vi "SS_FPGA_Drop1_all_in_v3.vi"() -> ()   [LabVIEW 2016]
uses:
  <vilib>/rvi/Emulation/niFpgaGetClockAttributes.vi
  <vilib>/rvi/Emulation/niFpgaSctlEmulationGetInTimedLoop.vi
  <vilib>/rvi/Emulation/niFpgaEmulationReportErrorSimple.vi
  <vilib>/rvi/Emulation/niFpgaCriticalErrorInLSC.vi
  <vilib>/rvi/Emulation/niFpgaProcessEmulError.vi
  <vilib>/rvi/eio/common/nirviEmuTemplateMethod_errors.vi
  <vilib>/eio/EIONode/EIONode.xnode
  <vilib>/rvi/FXPMathLib/FxpMul/XNode/nifxpmath_Multiplier.xnode
  <vilib>/rvi/FXPMathLib/FxpAdd/XNode/nifxpmath_Add.xnode
  <vilib>/rvi/FXPMathLib/sim/FxpSim.dll
panel:
  in  "Tab Control":T1(tab)
  in  "Start Acquisition":bool
  out "Actual Duration (ms)":u32
  out "Number of Loop 1 Samples":i32
  in  "Scan Rate (mSec) Loop 1":u32 caption="Count(mSec)"
  in  "Reset":bool
  in  "FSIS Interlock":bool
  out "Raw Data In Mod 1":fxp<+,24,12>[](array[numeric])
  in  "offset mod 1":fxp<+,24,12>[](array[numeric])=[0.0, 0.0, 0.0, 0.0, 0.0, 0.0, 0.0, 0.0, 0.0, 0.0, 0.0, 0.0, 0.0, 0.0, 0.0, 0.0]
  in  "cal mod 1":fxp<+,24,12>[](array[numeric])=[10.0, 10.0, 10.0, 10.0, 10.0, 10.0, 10.0, 10.0, 10.0, 10.0, 10.0, 10.0, 10.0, 10.0, 10.0, 10.0]
  out "Cal value out Mod 1":fxp<+,24,12>[](array[numeric]) format="%.16g"
  out "PTF - No Operations Mod 1":bool[](array[boolean])
  in  "lower limit \nNOOP mod 1":fxp<+,24,12>[](array[numeric])=[0.0, 0.0, 0.0, 0.0, 0.0, 0.0, 0.0, 0.0, 0.0, 0.0, 0.0, 0.0, 0.0, 0.0, 0.0, 0.0]
  in  "upper limit \nOKOP mod 1":fxp<+,24,12>[](array[numeric])=[0.0, 0.0, 0.0, 0.0, 0.0, 0.0, 0.0, 0.0, 0.0, 0.0, 0.0, 0.0, 0.0, 0.0, 0.0, 0.0]
  out "PTF - Warning Mod 1":bool[](array[boolean])
  in  "NOOPS Fault Filter mod 1":u16[](array[numeric])=[0, 0, 0, 0, 0, 0, 0, 0, 0, 0, 0, 0, 0, 0, 0, 0]
  out "Raw Data In Mod 2":fxp<+,24,12>[](array[numeric]) format="%.27g"
  in  "offset mod 2":fxp<+,24,12>[](array[numeric])=[0.0, 0.0, 0.0, 0.0, 0.0, 0.0, 0.0, 0.0, 0.0, 0.0, 0.0, 0.0, 0.0, 0.0, 0.0, 0.0]
  in  "cal mod 2":fxp<+,24,12>[](array[numeric])=[0.0, 0.0, 0.0, 0.0, 0.0, 0.0, 0.0, 0.0, 0.0, 0.0, 0.0, 0.0, 0.0, 0.0, 0.0, 0.0]
  out "PTF - No Operations Mod 2":bool[](array[boolean])
  in  "lower limit \nNOOP mod 2":fxp<+,24,12>[](array[numeric])=[0.0, 0.0, 0.0, 0.0, 0.0, 0.0, 0.0, 0.0, 0.0, 0.0, 0.0, 0.0, 0.0, 0.0, 0.0, 0.0]
  in  "upper limit \nOKOP mod 2":fxp<+,24,12>[](array[numeric])=[0.0, 0.0, 0.0, 0.0, 0.0, 0.0, 0.0, 0.0, 0.0, 0.0, 0.0, 0.0, 0.0, 0.0, 0.0, 0.0]
  out "Cal value out Mod 2":fxp<+,24,12>[](array[numeric])
  out "PTF - Warning Mod 2":bool[](array[boolean])
  in  "NOOPS Fault Filter mod 2":u16[](array[numeric])=[0, 0, 0, 0, 0, 0, 0, 0, 0, 0, 0, 0, 0, 0, 0, 0]
  out "Raw Data In Mod 3":fxp<+,24,12>[](array[numeric]) format="%.27g"
  in  "cal mod 3":fxp<+,24,12>[](array[numeric])=[0.0, 0.0, 0.0, 0.0, 0.0, 0.0, 0.0, 0.0, 0.0, 0.0, 0.0, 0.0, 0.0, 0.0, 0.0, 0.0]
  in  "offset mod 3":fxp<+,24,12>[](array[numeric])=[0.0, 0.0, 0.0, 0.0, 0.0, 0.0, 0.0, 0.0, 0.0, 0.0, 0.0, 0.0, 0.0, 0.0, 0.0, 0.0]
  out "PTF - No Operations Mod 3":bool[](array[boolean])
  in  "lower limit\nNOOP mod 3":fxp<+,24,12>[](array[numeric])=[0.0, 0.0, 0.0, 0.0, 0.0, 0.0, 0.0, 0.0, 0.0, 0.0, 0.0, 0.0, 0.0, 0.0, 0.0, 0.0]
  in  "upper limit\nOKOP mod 3":fxp<+,24,12>[](array[numeric])=[0.0, 0.0, 0.0, 0.0, 0.0, 0.0, 0.0, 0.0, 0.0, 0.0, 0.0, 0.0, 0.0, 0.0, 0.0, 0.0]
  out "PTF - Warning Mod 3":bool[](array[boolean])
  out "Cal value out Mod 3":fxp<+,24,12>[](array[numeric])
  in  "NOOPS Fault Filter mod 3":u16[](array[numeric])=[0, 0, 0, 0, 0, 0, 0, 0, 0, 0, 0, 0, 0, 0, 0, 0]
  out "Raw Data In Mod 4":fxp<+,24,12>[](array[numeric]) format="%.27g"
  out "Raw Data In Mod 5":fxp<+,24,12>[](array[numeric]) format="%.27g"
  out "Raw Data In Mod 6":bool[](array[boolean])
  out "Trigger from Trigger Card (SYNC and ASYNC) (Euro1Slot15)":bool
  out "Main Trigger In":bool
  out "SYNC/ASYNC":bool
  out "Beam Prepare":bool
  out "Override":bool
  out "320 Open":bool
  out "320  Closed":bool
  out "400 Open":bool
  out "400 Open Closed":bool
  out "Calorimeter Left Gate Open":bool
  out "Calorimeter Left Gate Closed":bool
  out "320  Bypass Open":bool
  out "320 Bypass Closed":bool
  out "Calorimeter Right Gate Closed":bool
  out "HV Area Water":bool
  out "MAST Area Air":bool
  out "Calorimeter Right Gate Open":bool
  in  "Control FBIS 1kHZ":bool
  # "CHANNEL ID"
  # "1"
  # "SS Source Body Flow\n\nSS Source Body Temperature\n\nSS Grid 1 Flow\n\nSS Grid 1 Temperature\n\nSS Grid 2 Flow\n\nSS Grid 2 Temperature\n\nSS Grid 3 Flow\n\nSS Grid 3 Temperature\n\nSS Grid 4/1st Stage Neutraliser Flow\n\nSS Grid 4/1st Stage Neutraliser Temperature\n\nSS 2nd Stage Neutraliser Flow\n\nSS 2nd Stage Neutraliser Temperature\n\nSS PINI Backplate Flow\n\nSS PINI Backplate Temperature\n\nSS Duct Scraper Flow\n\nSS Duct Scraper Temperature"
  # "2"
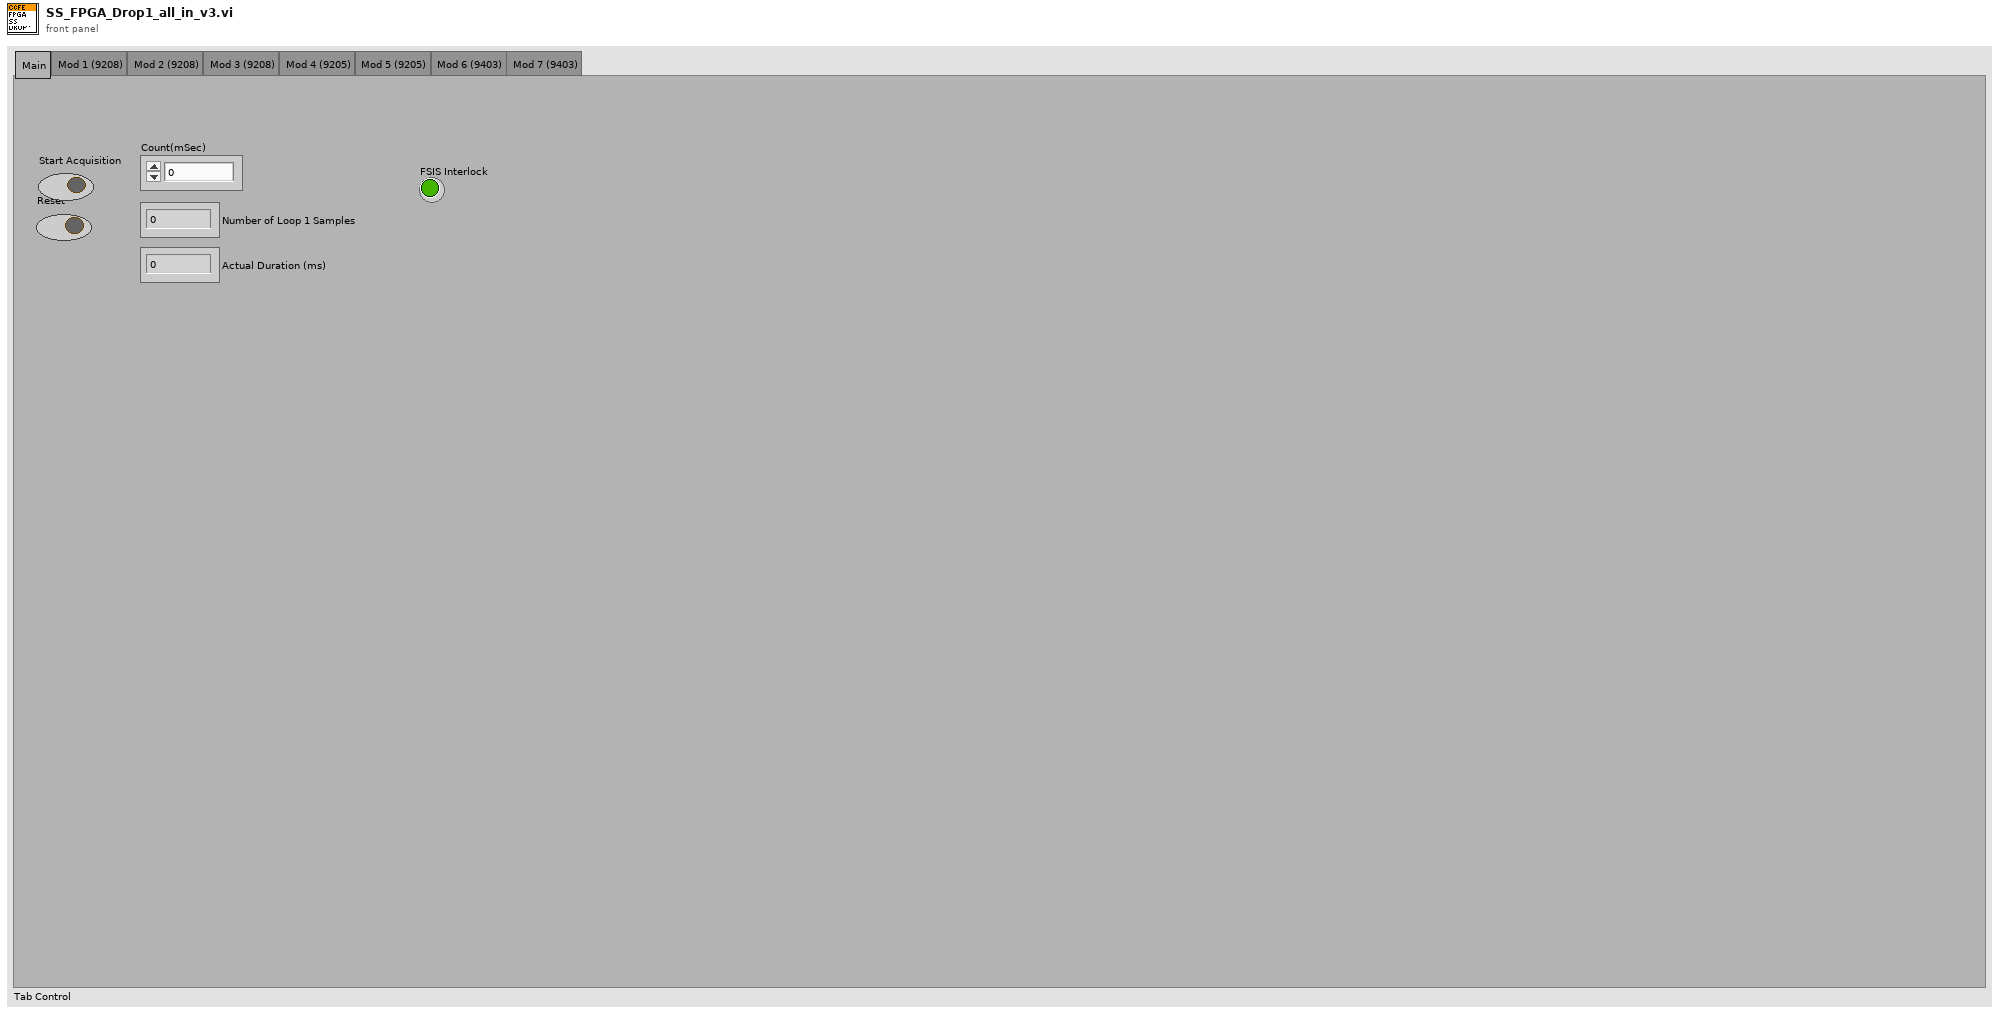
[diagram p1: front panel]
types:
  T1 = enum32{"Main", "Mod 1 (9208)", "Mod 2 (9208)", "Mod 3 (9208)", "Mod 4 (9205)", "Mod 5 (9205)", "Mod 6 (9403)", "Mod 7 (9403)"}
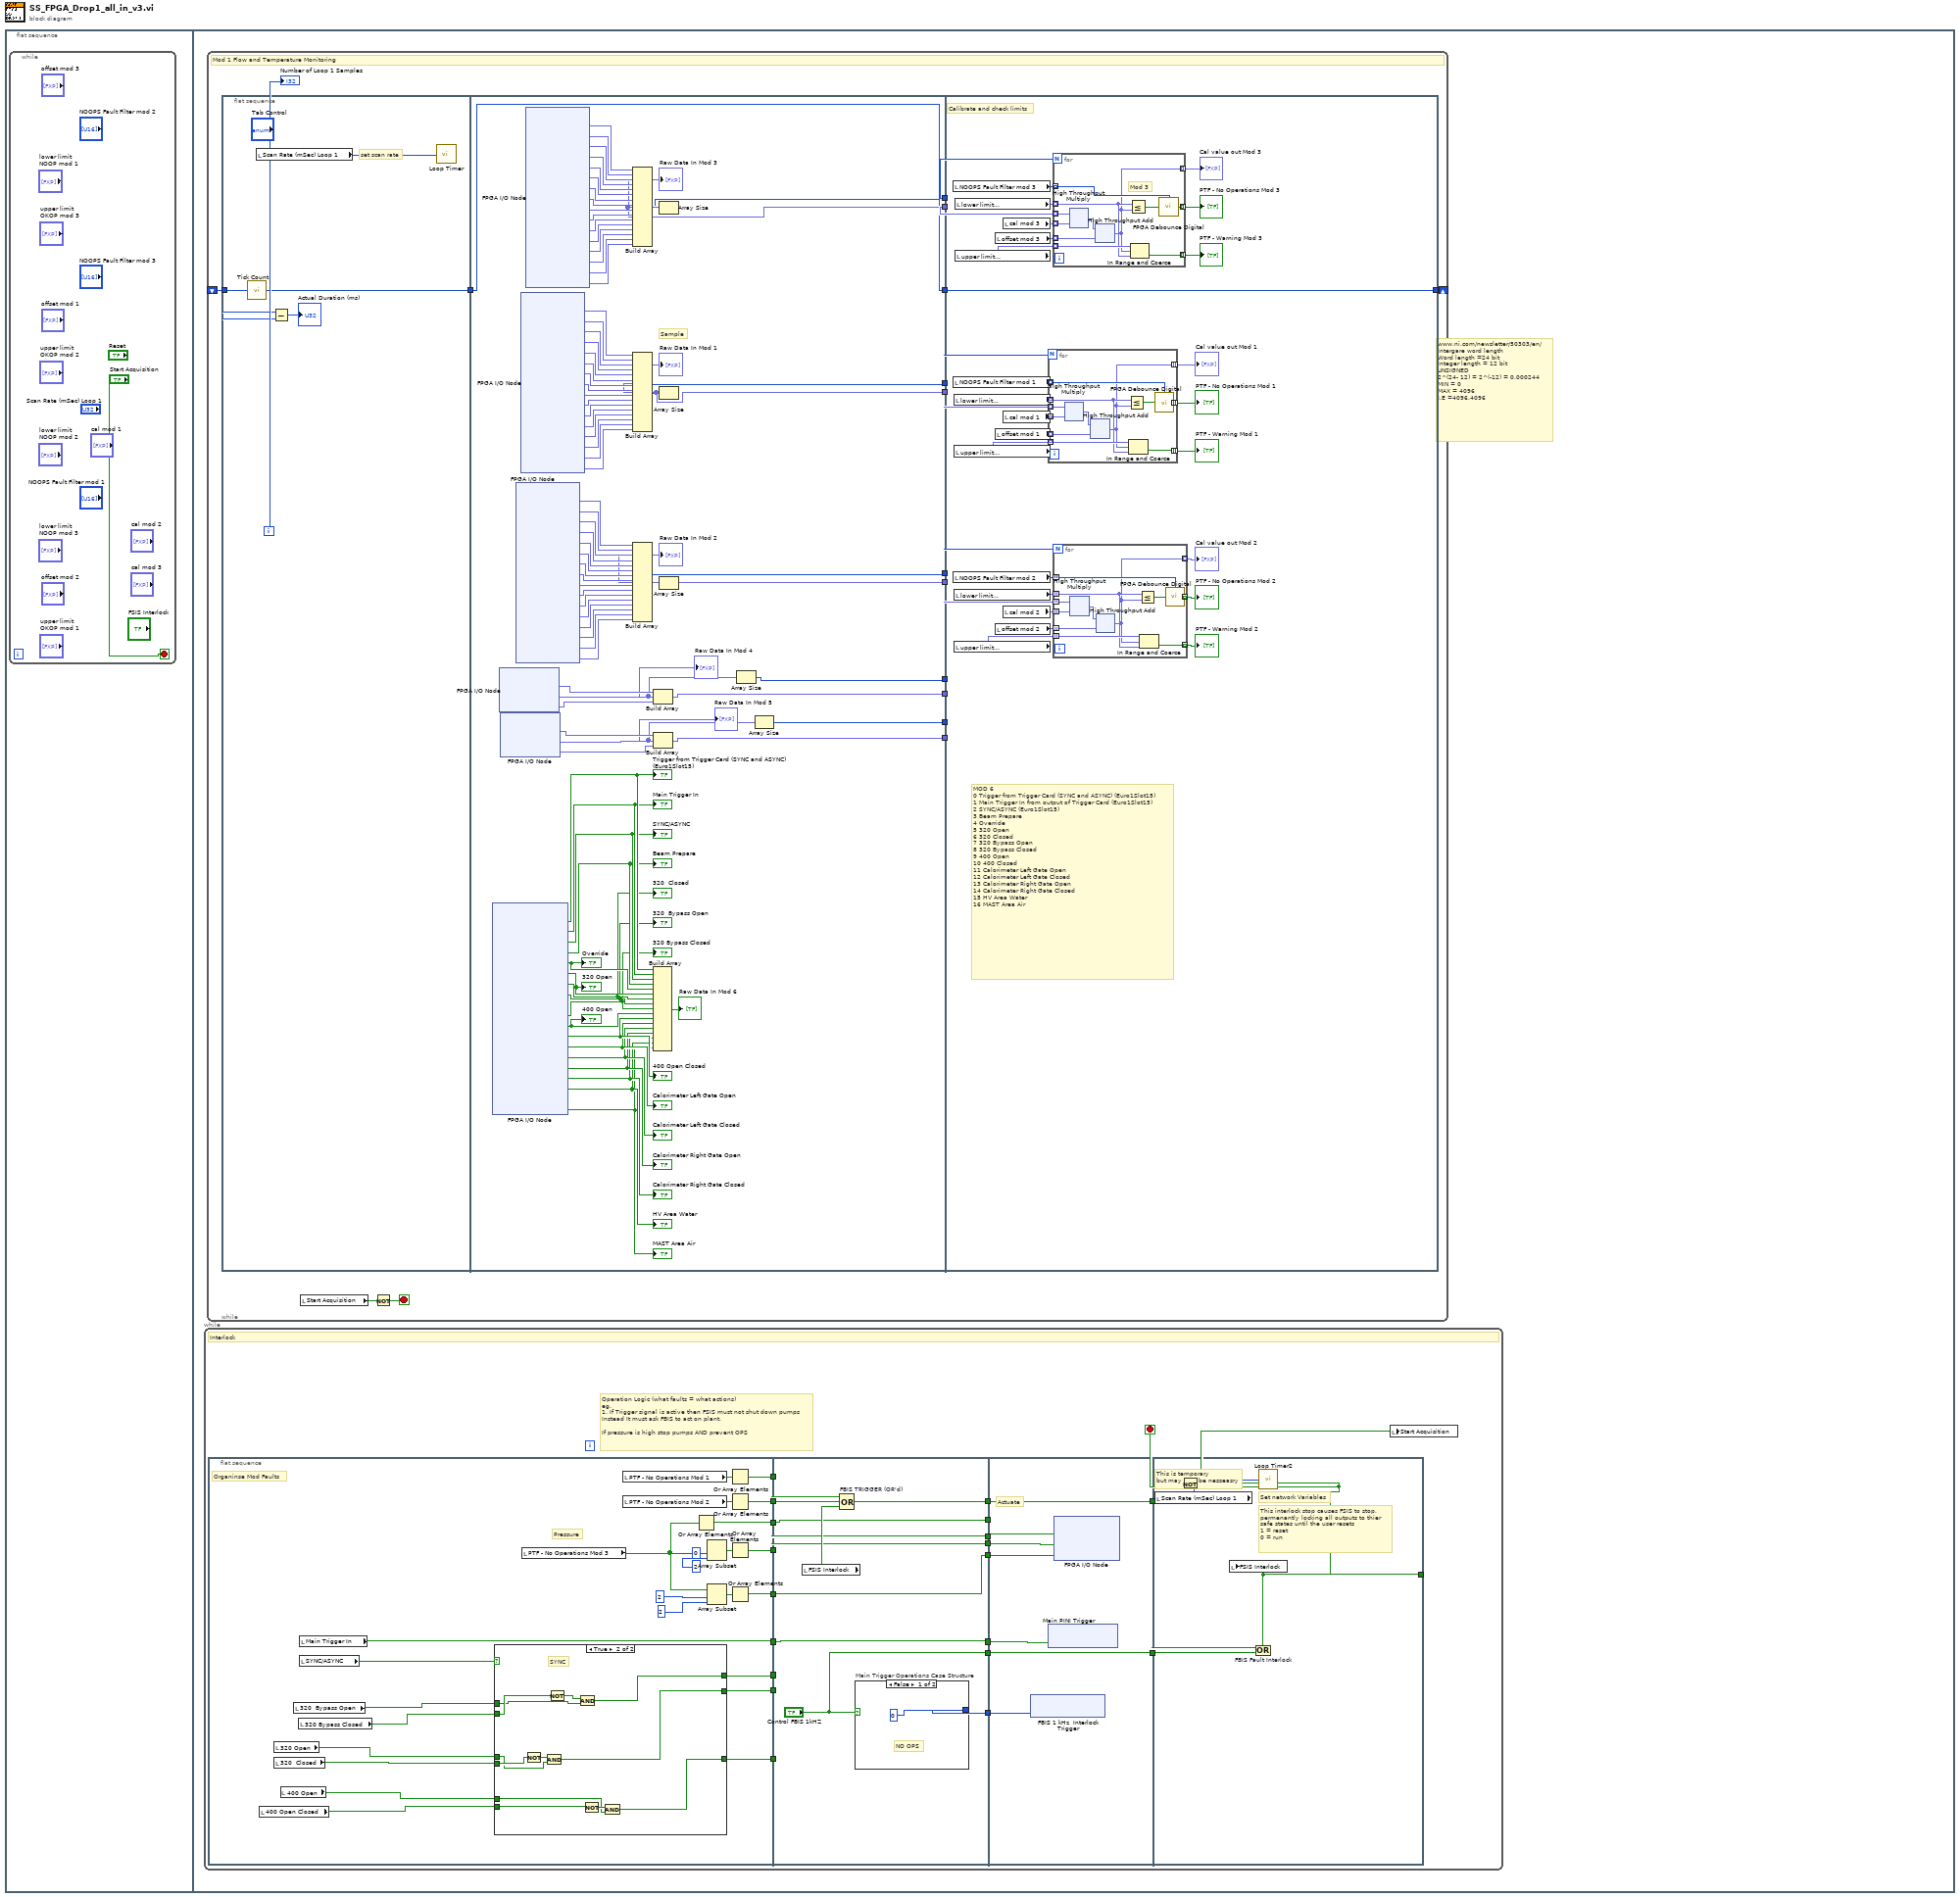
[diagram p0: block diagram]
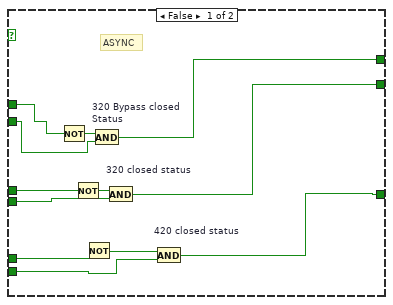
[diagram p2: hidden frame]
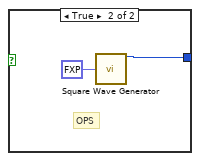
[diagram p3: hidden frame]
diagram:
  n1 = flat-sequence {
    frame #0 {
      n2 = while {
        stop <- "Start Acquisition" stop-if-true
      }
    }
    frame #1 {
      # "www.ni.com/newsletter/50303/en/\nIntergare word length \nWord length =24 bit\nInteger length = 12 bit\nUNSIGNED\n2^(24- 12) = 2^(-12) = 0.000244\nMIN = 0 \nMAX = 4096\nI.E =4096.4096"
      n3 = while {
        stop <- w18 stop-if-true
        # "Operation Logic (what faults = what actions)\neg.\n1. If Trigger signal is active then FSIS must not shut down pumps\nInstead It must ask FBIS to act on plant.\n\nIf pressure is high stop pumps AND prevent OPS"
        # "Interlock"
        n4 = flat-sequence {
          tunnel: [w47] -> w21
          tunnel: [w46] -> w16
          tunnel: [w43] -> w15
          tunnel: [w39] -> w13
          tunnel: [w35] -> w11
          tunnel: [w26] -> w10
          tunnel: [w25] -> w9
          tunnel: [w24] -> w8
          tunnel: [w23] -> w6
          tunnel: [w77] -> w22
          tunnel: w21 -> [w80]
          tunnel: [w80] -> w17
          tunnel: w16 -> [w79]
          tunnel: w15 -> [w78]
          tunnel: [w76] -> w14
          tunnel: w13 -> [w76]
          tunnel: [w74] -> w12
          tunnel: w11 -> [w74]
          tunnel: w10 -> [_]
          tunnel: w9 -> [_]
          tunnel: w8 -> [_]
          tunnel: [w75] -> w7
          tunnel: w6 -> [w73]
          tunnel: [w74] -> w5
          tunnel: [w73] -> w4
          tunnel: ["Control FBIS 1kHZ"] -> w3
          tunnel: w22 -> [w91]
          tunnel: [w91] -> w20
          tunnel: w17 -> [_]
          tunnel: w14 -> [w90]
          tunnel: w12 -> [w89]
          tunnel: w7 -> [w87]
          tunnel: w5 -> [w88]
          tunnel: w4 -> [w86]
          tunnel: w3 -> [w85]
          tunnel: [w85] -> w2
          tunnel: w20 -> [w94]
          tunnel: [w93] -> w18
          tunnel: w2 -> [w92]
          frame #0 {
            # "Pressure"
            # "Organinse Mod Faults"
            n5 = local read "400 Open Closed"() -> (w30:bool)
            n6 = local read "320 Open"() -> (w27:bool)
            n7 = local read "320  Closed"() -> (w28:bool)
            n8 = local read "400 Open"() -> (w31:bool)
            n9 = local read "320  Bypass Open"() -> (w32:bool)
            n10 = local read "320 Bypass Closed"() -> (w29:bool)
            n11 = local read "Main Trigger In"() -> (w23:bool)
            n12 = local read "SYNC/ASYNC"() -> (w33:bool)
            n13 = case shown="True" w33 {
              tunnel: w32 -> [w59 w67]
              tunnel: w31 -> [w51 w65]
              tunnel: w30 -> [w55 w66]
              tunnel: w29 -> [w54 w68]
              tunnel: w28 -> [w53 w64]
              tunnel: w27 -> [w52 w63]
              tunnel: [w48 w60] -> w24
              tunnel: [w50 w61] -> w25
              tunnel: [w49 w62] -> w26
              frame False {
                # "ASYNC"
                n14 = Not(x=w59) -> (.not. x?=w58:bool)
                n15 = Not(x=w52) -> (.not. x?=w57:bool)
                n16 = Not(x=w51) -> (.not. x?=w56:bool)
                n17 = And "320 Bypass closed Status"(x=w58, y=w54) -> (x .and. y?=w49:bool)
                n18 = And "320 closed status"(x=w57, y=w53) -> (x .and. y?=w50:bool)
                n19 = And "420 closed status"(x=w56, y=w55) -> (x .and. y?=w48:bool)
              }
              frame True {
                # "SYNC"
                n20 = Not(x=w64) -> (.not. x?=w69:bool)
                n21 = And(x=w69, y=w63) -> (x .and. y?=w61:bool)
                n22 = Not(x=w68) -> (.not. x?=w71:bool)
                n23 = And(x=w71, y=w67) -> (x .and. y?=w62:bool)
                n24 = Not(x=w66) -> (.not. x?=w70:bool)
                n25 = And(x=w70, y=w65) -> (x .and. y?=w60:bool)
              }
            }
            n26 = local read "PTF - No Operations Mod 3"() -> (w34:bool[])
            n27 = local read "PTF - No Operations Mod 1"() -> (w45:bool[])
            n28 = local read "PTF - No Operations Mod 2"() -> (w44:bool[])
            n29 = Or Array Elements(Boolean array=w34) -> (logical OR=w47:bool)
            n30 = Array Subset(array=w34, index=0, length=2) -> (w40:bool[])
            n31 = Array Subset(array=w34, index=2, length=2) -> (w36:bool[])
            n32 = Or Array Elements(Boolean array=w45) -> (logical OR=w46:bool)
            n33 = Or Array Elements(Boolean array=w44) -> (logical OR=w43:bool)
            n34 = Or Array Elements(Boolean array=w40) -> (logical OR=w39:bool)
            n35 = Or Array Elements(Boolean array=w36) -> (logical OR=w35:bool)
          }
          frame #1 {
            n36 = local read "FSIS Interlock"() -> (w81:bool)
            n37 = Compound Arithmetic op=OR "FBIS TRIGGER (OR'd)"(w79, w78, w81) -> (w77:bool)
            n38 = case "Main Trigger Operations Case Structure" shown="False" "Control FBIS 1kHZ" {
              tunnel: [u8 0 ("duty cycle (periods)") w83] -> w75
              frame False {
                # "NO OPS"
              }
              frame True {
                # "OPS"
                n39 = call "Square Wave Generator"("duty cycle (periods)"=fxp<+,32,0> 0.5) -> ("square wave out"=w83:i16)  [unwired: 14 in]
              }
            }
          }
          frame #2 {
            # "Actuate"
            n40 = xnode "FBIS 1 kHz  Interlock Trigger"("Mod7/DIO31:0"=w87) -> ()  [unwired: 1 in, 1 out]
            n41 = xnode "Main PINI Trigger"("Mod7/DIO17"=w86) -> ()  [unwired: 1 in, 1 out]
            n42 = xnode "FPGA I/O Node"("Mod7/DIO0"=w90, "Mod7/DIO1"=w89, "Mod7/DIO2"=w88) -> ()  [unwired: 3 in, 3 out]
          }
          frame #3 {
            # "This interlock stop causes FSIS to stop,\npermenantly locking all outputs to thier \nsafe states until the user resets\n1 = reset\n0 = run"
            # "This is temporary\nbut may also be nesseasry"
            # "Set network Variables"
            n43 = local read "Scan Rate (mSec) Loop 1"() -> (w95:u32)
            n44 = Compound Arithmetic op=OR "FBIS Fault Interlock"(w94, w92) -> (w93:bool)
            n45 = local write "FSIS Interlock"(w93) -> ()
            n46 = call "Loop Timer2"("Count(mSec)"=w95) -> ()  [unwired: 1 out]
          }
        }
        n47 = Not(x=w18) -> (.not. x?=w19:bool)
        n48 = local write "Start Acquisition"(w19) -> ()
      }
      n49 = while {
        shift-right: [w111] -> _
        shift-left: _ -> [w109]
        i -> [w112]
        stop <- w108 stop-if-true
        # "Mod 1 Flow and Temperature Monitoring"
        n50 = flat-sequence {
          tunnel: [w113] -> w110
          tunnel: w109 -> [w114]
          tunnel: w110 -> [w183]
          tunnel: [w183] -> w106
          tunnel: [w153] -> w105
          tunnel: [w149] -> w104
          tunnel: [w148] -> w103
          tunnel: [w146] -> w102
          tunnel: [w147] -> w101
          tunnel: [w145] -> w100
          tunnel: [w137] -> w99
          tunnel: [w136] -> w98
          tunnel: [w138] -> w97
          tunnel: [w135] -> w96
          tunnel: w106 -> [w230]
          tunnel: w105 -> [w219]
          tunnel: w104 -> [w218]
          tunnel: w103 -> [w229]
          tunnel: w102 -> [w224]
          tunnel: w101 -> [w217]
          tunnel: w100 -> [w216]
          tunnel: [w230] -> w111
          tunnel: w99 -> [_]
          tunnel: w98 -> [_]
          tunnel: w97 -> [_]
          tunnel: w96 -> [_]
          frame #0 {
            # "set scan rate"
            n51 = call "Tick Count"() -> ("Tick Count(mSec)"=w113:u32)
            n52 = local read "Scan Rate (mSec) Loop 1"() -> (w116:u32)
            n53 = Subtract(x=w113, y=w114) -> (x-y=→"Actual Duration (ms)":u32)
            n54 = call "Loop Timer"("Count(mSec)"=w116) -> ()  [unwired: 1 out]
          }
          frame #1 {
            # "Sample"
            n55 = xnode "FPGA I/O Node"() -> ("Mod6/DIO0"=w144:bool, "Mod6/DIO1"=w132:bool, "Mod6/DIO2"=w131:bool, "Mod6/DIO3"=w130:bool, "Mod6/DIO4"=w129:bool, "Mod6/DIO5"=w128:bool, "Mod6/DIO6"=w127:bool, "Mod6/DIO7"=w126:bool, "Mod6/DIO8"=w125:bool, "Mod6/DIO9"=w124:bool, "Mod6/DIO10"=w123:bool, "Mod6/DIO11"=w122:bool, "Mod6/DIO12"=w121:bool, "Mod6/DIO13"=w120:bool, "Mod6/DIO14"=w119:bool, "Mod6/DIO15"=w118:bool, "Mod6/DIO16"=w117:bool)  [unwired: 19 in, 21 out]
            "Trigger from Trigger Card (SYNC and ASYNC) (Euro1Slot15)" <- w144
            "Main Trigger In" <- w132
            "SYNC/ASYNC" <- w131
            "Beam Prepare" <- w130
            "Override" <- w129
            "320 Open" <- w128
            "320  Closed" <- w127
            "400 Open" <- w124
            "400 Open Closed" <- w123
            "Calorimeter Left Gate Open" <- w122
            "Calorimeter Left Gate Closed" <- w121
            "320  Bypass Open" <- w126
            "320 Bypass Closed" <- w125
            "Calorimeter Right Gate Closed" <- w119
            "HV Area Water" <- w118
            "MAST Area Air" <- w117
            "Calorimeter Right Gate Open" <- w120
            n56 = xnode "FPGA I/O Node"() -> ("Mod4/AI0"=w142:fxp<+/-,24,-4>, "Mod4/AI1"=w141:fxp<+/-,24,-4>, "Mod4/AI2"=w134:fxp<+/-,24,-4>)  [unwired: 3 in, 3 out]
            n57 = xnode "FPGA I/O Node"() -> ("Mod5/AI0"=w140:fxp<+/-,26,5>, "Mod5/AI1"=w139:fxp<+/-,26,5>, "Mod5/AI2"=w133:fxp<+/-,26,5>)  [unwired: 3 in, 3 out]
            n58 = xnode "FPGA I/O Node"() -> ("Mod2/AI0"=w154:fxp<+/-,24,-4>, "Mod2/AI1"=w155:fxp<+/-,24,-4>, "Mod2/AI2"=w156:fxp<+/-,24,-4>, "Mod2/AI3"=w157:fxp<+/-,24,-4>, "Mod2/AI4"=w158:fxp<+/-,24,-4>, "Mod2/AI5"=w159:fxp<+/-,24,-4>, "Mod2/AI6"=w160:fxp<+/-,24,-4>, "Mod2/AI7"=w161:fxp<+/-,24,-4>, "Mod2/AI8"=w162:fxp<+/-,24,-4>, "Mod2/AI9"=w163:fxp<+/-,24,-4>, "Mod2/AI10"=w164:fxp<+/-,24,-4>, "Mod2/AI11"=w165:fxp<+/-,24,-4>, "Mod2/AI12"=w166:fxp<+/-,24,-4>, "Mod2/AI13"=w167:fxp<+/-,24,-4>, "Mod2/AI14"=w168:fxp<+/-,24,-4>, "Mod2/AI15"=w169:fxp<+/-,24,-4>)  [unwired: 16 in, 16 out]
            n59 = xnode "FPGA I/O Node"() -> ("Mod1/AI0"=w199:fxp<+/-,24,-4>, "Mod1/AI1"=w198:fxp<+/-,24,-4>, "Mod1/AI2"=w197:fxp<+/-,24,-4>, "Mod1/AI3"=w196:fxp<+/-,24,-4>, "Mod1/AI4"=w195:fxp<+/-,24,-4>, "Mod1/AI5"=w194:fxp<+/-,24,-4>, "Mod1/AI6"=w193:fxp<+/-,24,-4>, "Mod1/AI7"=w192:fxp<+/-,24,-4>, "Mod1/AI8"=w191:fxp<+/-,24,-4>, "Mod1/AI9"=w190:fxp<+/-,24,-4>, "Mod1/AI10"=w189:fxp<+/-,24,-4>, "Mod1/AI11"=w188:fxp<+/-,24,-4>, "Mod1/AI12"=w187:fxp<+/-,24,-4>, "Mod1/AI13"=w186:fxp<+/-,24,-4>, "Mod1/AI14"=w185:fxp<+/-,24,-4>, "Mod1/AI15"=w184:fxp<+/-,24,-4>)  [unwired: 16 in, 16 out]
            n60 = xnode "FPGA I/O Node"() -> ("Mod3/AI0"=w182:fxp<+/-,24,-4>, "Mod3/AI1"=w181:fxp<+/-,24,-4>, "Mod3/AI2"=w180:fxp<+/-,24,-4>, "Mod3/AI3"=w179:fxp<+/-,24,-4>, "Mod3/AI4"=w178:fxp<+/-,24,-4>, "Mod3/AI5"=w177:fxp<+/-,24,-4>, "Mod3/AI6"=w176:fxp<+/-,24,-4>, "Mod3/AI7"=w175:fxp<+/-,24,-4>, "Mod3/AI8"=w174:fxp<+/-,24,-4>, "Mod3/AI9"=w173:fxp<+/-,24,-4>, "Mod3/AI10"=w172:fxp<+/-,24,-4>, "Mod3/AI11"=w171:fxp<+/-,24,-4>, "Mod3/AI12"=w170:fxp<+/-,24,-4>, "Mod3/AI13"=w152:fxp<+/-,24,-4>, "Mod3/AI14"=w151:fxp<+/-,24,-4>, "Mod3/AI15"=w150:fxp<+/-,24,-4>)  [unwired: 16 in, 16 out]
            n61 = Build Array(w182, w181, w180, w179, w178, w177, w176, w175, w174, w173, w172, w171, w170, w152, w151, w150) -> (w146:fxp<+/-,24,-4>[])
            "Raw Data In Mod 3" <- w146
            n62 = Build Array(w199, w198, w197, w196, w195, w194, w193, w192, w191, w190, w189, w188, w187, w186, w185, w184) -> (w149:fxp<+/-,24,-4>[])
            "Raw Data In Mod 1" <- w149
            n63 = Build Array(w154, w155, w156, w157, w158, w159, w160, w161, w162, w163, w164, w165, w166, w167, w168, w169) -> (w148:fxp<+/-,24,-4>[])
            "Raw Data In Mod 2" <- w148
            n64 = Build Array(w144, w132, w131, w130, w129, w128, w127, w126, w125, w124, w123, w122, w121, w120, w119, w118, w117) -> (→"Raw Data In Mod 6":bool[])
            n65 = Build Array(w142, w141, w134) -> (w137:fxp<+/-,24,-4>[])
            "Raw Data In Mod 4" <- w137
            n66 = Build Array(w140, w139, w133) -> (w136:fxp<+/-,26,5>[])
            "Raw Data In Mod 5" <- w136
            n67 = Array Size(array=w146) -> (size(s)=w145:i32)
            n68 = Array Size(array=w149) -> (size(s)=w153:i32)
            n69 = Array Size(array=w148) -> (size(s)=w147:i32)
            n70 = Array Size(array=w137) -> (size(s)=w138:i32)
            n71 = Array Size(array=w136) -> (size(s)=w135:i32)
          }
          frame #2 {
            # "MOD 6\n0\tTrigger from Trigger Card (SYNC and ASYNC) (Euro1Slot15)\n1\tMain Trigger In from output of Trigger Card (Euro1Slot15)\n2\tSYNC/ASYNC (Euro1Slot15)\n3\tBeam Prepare\n4\tOverride\n5\t320 Open\n6\t320 Closed\n7\t320 Bypass Open\n8\t320 Bypass Closed\n9\t400 Open \n10\t400 Closed\n11\tCalorimeter Left Gate Open\n12\tCalorimeter Left Gate Closed\n13\tCalorimeter Right Gate Open\n14\tCalorimeter Right Gate Closed\n15\tHV Area Water\n16\tMAST Area Air"
            # "Calibrate and check limits"
            n72 = local read "NOOPS Fault Filter mod 3"() -> (w202:u16[])
            n73 = local read "NOOPS Fault Filter mod 1"() -> (w203:u16[])
            n74 = local read "NOOPS Fault Filter mod 2"() -> (w201:u16[])
            n75 = local read "lower limit \nNOOP mod 1"() -> (w215:fxp<+,24,12>[])
            n76 = local read "upper limit \nOKOP mod 1"() -> (w214:fxp<+,24,12>[])
            n77 = local read "lower limit \nNOOP mod 2"() -> (w225:fxp<+,24,12>[])
            n78 = local read "upper limit \nOKOP mod 2"() -> (w226:fxp<+,24,12>[])
            n79 = local read "lower limit\nNOOP mod 3"() -> (w221:fxp<+,24,12>[])
            n80 = local read "upper limit\nOKOP mod 3"() -> (w220:fxp<+,24,12>[])
            n81 = local read "offset mod 3"() -> (w222:fxp<+,24,12>[])
            n82 = local read "offset mod 1"() -> (w212:fxp<+,24,12>[])
            n83 = local read "offset mod 2"() -> (w228:fxp<+,24,12>[])
            n84 = local read "cal mod 3"() -> (w223:fxp<+,24,12>[])
            n85 = local read "cal mod 1"() -> (w213:fxp<+,24,12>[])
            n86 = local read "cal mod 2"() -> (w227:fxp<+,24,12>[])
            n87 = for {
              N: w219 -> [_]
              tunnel: w213 -> [w234] mode=indexing
              tunnel: w212 -> [w233] mode=indexing
              tunnel: w218 -> [w232] mode=indexing
              tunnel: w214 -> [w241] mode=indexing
              tunnel: w215 -> [w240] mode=indexing
              tunnel: [w238] -> w207 mode=indexing
              tunnel: [w237] -> w206 mode=indexing
              tunnel: w203 -> [w236] mode=indexing
              tunnel: [w231] -> w200 mode=indexing
              n88 = xnode ("High Throughput Multiply")("x"=w232, "y"=w234) -> ("x*y"=w235:fxp<+,24,12>)
              n89 = xnode ("High Throughput Add")("x"=w235, "y"=w233) -> ("x+y"=w231:fxp<+,24,12>)
              n90 = Less Or Equal?(x=w240, y=w231) -> (x <= y?=w239:bool)
              n91 = In Range and Coerce(upper limit=w241, x=w231, lower limit=w240) -> (In Range?=w237:bool)  [unwired: 1 out]
              n92 = call "FPGA Debounce Digital.vi"("Input Signal"=w239, "Cycles to Filter"=w236) -> ("Output Filtered Signal"=w238:bool)
            }
            "Cal value out Mod 1" <- w200
            "PTF - No Operations Mod 1" <- w207
            "PTF - Warning Mod 1" <- w206
            n93 = for {
              N: w216 -> [_]
              tunnel: w223 -> [w244] mode=indexing
              tunnel: w222 -> [w246] mode=indexing
              tunnel: w224 -> [w245] mode=indexing
              tunnel: [w242] -> w211 mode=indexing
              tunnel: w220 -> [w251] mode=indexing
              tunnel: w221 -> [w250] mode=indexing
              tunnel: [w252] -> w209 mode=indexing
              tunnel: [w248] -> w208 mode=indexing
              tunnel: w202 -> [w247] mode=indexing
              # "Mod 3"
              n94 = xnode ("High Throughput Multiply")("x"=w245, "y"=w244) -> ("x*y"=w243:fxp<+,24,12>)
              n95 = xnode ("High Throughput Add")("x"=w243, "y"=w246) -> ("x+y"=w242:fxp<+,24,12>)
              n96 = Less Or Equal?(x=w250, y=w242) -> (x <= y?=w249:bool)
              n97 = In Range and Coerce(upper limit=w251, x=w242, lower limit=w250) -> (In Range?=w252:bool)  [unwired: 1 out]
              n98 = call "FPGA Debounce Digital.vi"("Input Signal"=w249, "Cycles to Filter"=w247) -> ("Output Filtered Signal"=w248:bool)
            }
            "Cal value out Mod 3" <- w211
            "PTF - No Operations Mod 3" <- w208
            "PTF - Warning Mod 3" <- w209
            n99 = for {
              N: w217 -> [_]
              tunnel: w227 -> [w257] mode=indexing
              tunnel: w228 -> [w255] mode=indexing
              tunnel: w229 -> [w256] mode=indexing
              tunnel: [w253] -> w210 mode=indexing
              tunnel: w226 -> [w262] mode=indexing
              tunnel: w225 -> [w261] mode=indexing
              tunnel: [w263] -> w204 mode=indexing
              tunnel: [w259] -> w205 mode=indexing
              tunnel: w201 -> [w258] mode=indexing
              n100 = xnode ("High Throughput Multiply")("x"=w256, "y"=w257) -> ("x*y"=w254:fxp<+,24,12>)
              n101 = xnode ("High Throughput Add")("x"=w254, "y"=w255) -> ("x+y"=w253:fxp<+,24,12>)
              n102 = Less Or Equal?(x=w261, y=w253) -> (x <= y?=w260:bool)
              n103 = In Range and Coerce(upper limit=w262, x=w253, lower limit=w261) -> (In Range?=w263:bool)  [unwired: 1 out]
              n104 = call "FPGA Debounce Digital.vi"("Input Signal"=w260, "Cycles to Filter"=w258) -> ("Output Filtered Signal"=w259:bool)
            }
            "Cal value out Mod 2" <- w210
            "PTF - No Operations Mod 2" <- w205
            "PTF - Warning Mod 2" <- w204
          }
        }
        n105 = local read "Start Acquisition"() -> (w107:bool)
        n106 = Not(x=w107) -> (.not. x?=w108:bool)
        "Number of Loop 1 Samples" <- w112
      }
    }
  }
